vi "CSDB_Transfer.disable controls.vi"(2 "error in (no error)":errorcluster, 3 "on / off":bool, 4 "Tab Control":refnum<vi>) -> (0 "error out":errorcluster)   [LabVIEW 2014, in "CSDB_Transfer.lvlib"]
doc: "En/Disables all fp controls"
uses:
  CSDB_Transfer.lvlib
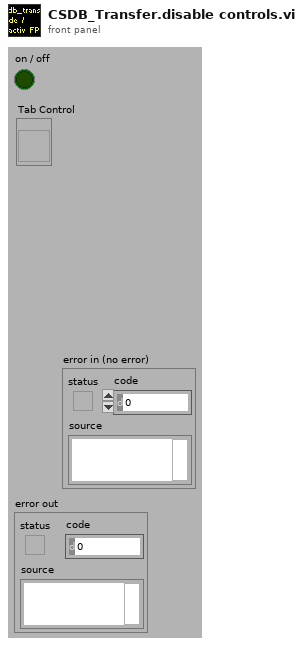
[diagram p1: front panel]
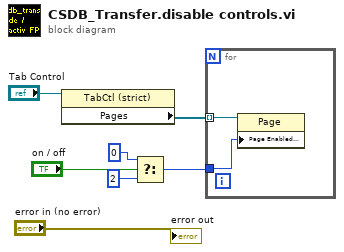
[diagram p0: block diagram]
diagram:
  n1 = property class="TabCtl (strict)"(reference="Tab Control") -> ("Pages"=w7:refnum<vi>[])  [unwired: 1 in, 2 out]
  n2 = Select(t=0, s="on / off", f=2) -> (s? t:f=w5:i32)
  n3 = for {
    tunnel: w7 -> [w9] mode=indexing
    tunnel: w5 -> [w8]
    n4 = property class="Page"(reference=w9, "Page Enabled State"=w8) -> ()  [unwired: 1 in, 2 out]
  }
  "error out" <- "error in (no error)"
